vi "DancingLED.vi"() -> ()   [LabVIEW 2020]
uses:
  DancingLEDEnum.ctl
  bcbb1c2d-c491-4427-a344-9a07431e1d3e.vi
  939999a5-51db-4c4a-bf67-1753f00f95a7.vi
  fbb08f2d-998a-4061-bdb6-f44989c1556d.vi
  5b1967e0-138d-40db-84bc-8d854150fb75.vi
  e170c4a2-dbbe-475a-b394-96526eb2ee03.vi
  <vilib>/ErrorRing/Error Ring.xnode
panel:
  out "5":bool[](array[boolean])
  out "4":bool[](array[boolean])
  out "3":bool[](array[boolean])
  out "2":bool[](array[boolean])
  out "1":bool[](array[boolean])
  in  "Switch":bool
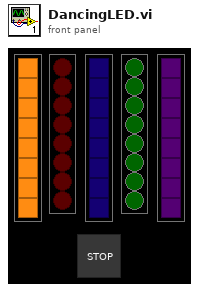
[diagram p1: front panel]
types:
  T1 = typedef "DancingLEDEnum.ctl" = enum16{"IDLE", "CONTROL", "UIInit", "DataUpdate", "UPDATE", "EXIT"}
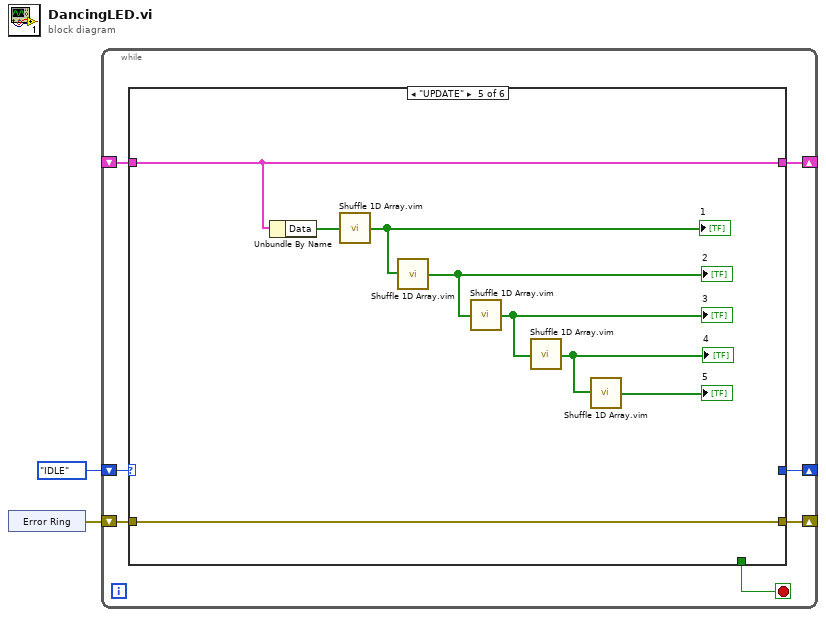
[diagram p0: block diagram]
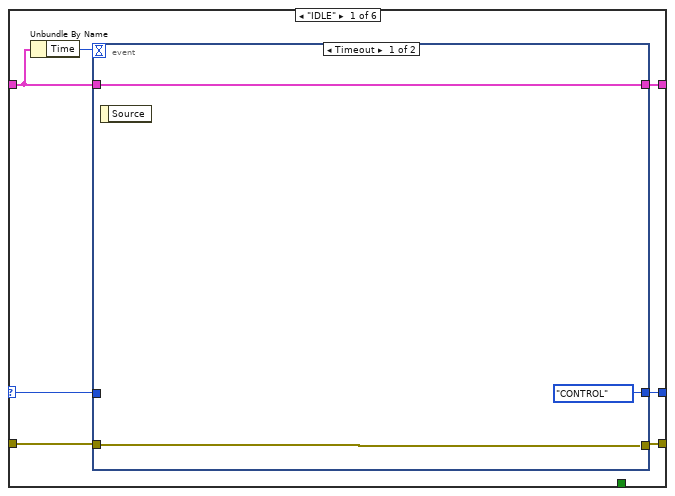
[diagram p2: hidden frame]
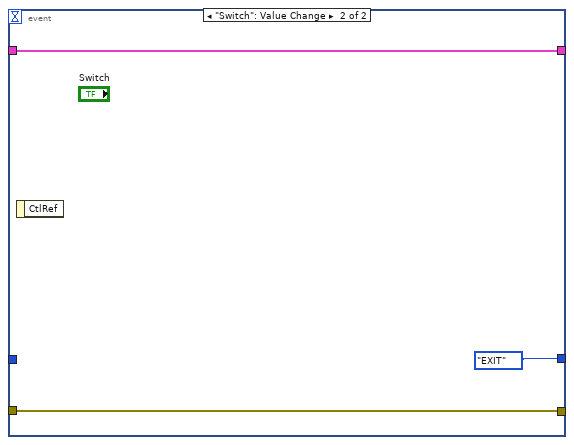
[diagram p3: hidden frame]
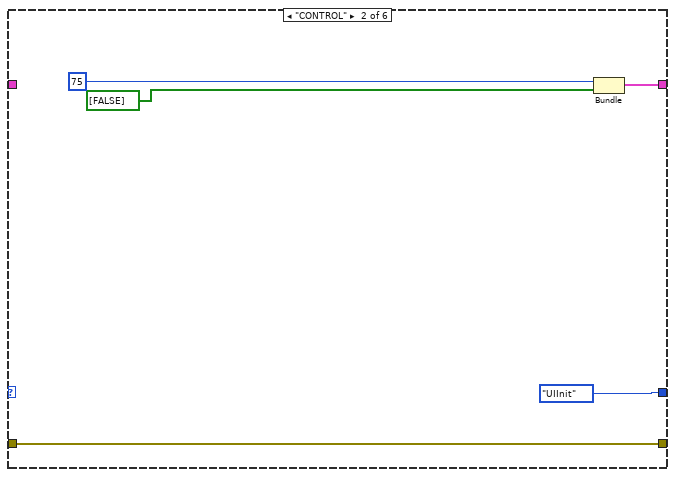
[diagram p4: hidden frame]
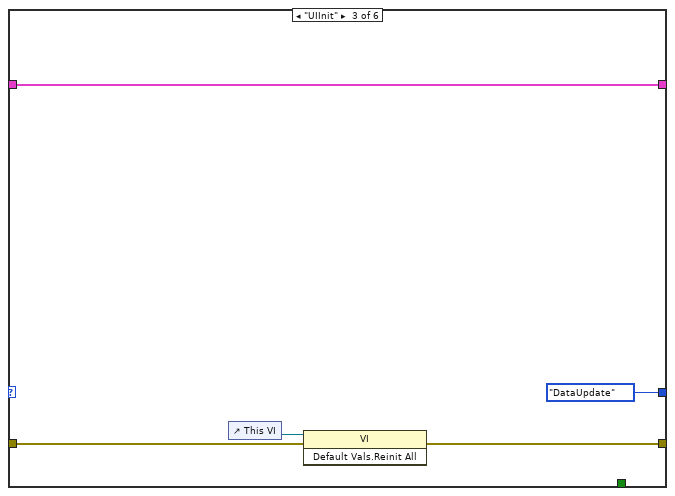
[diagram p5: hidden frame]
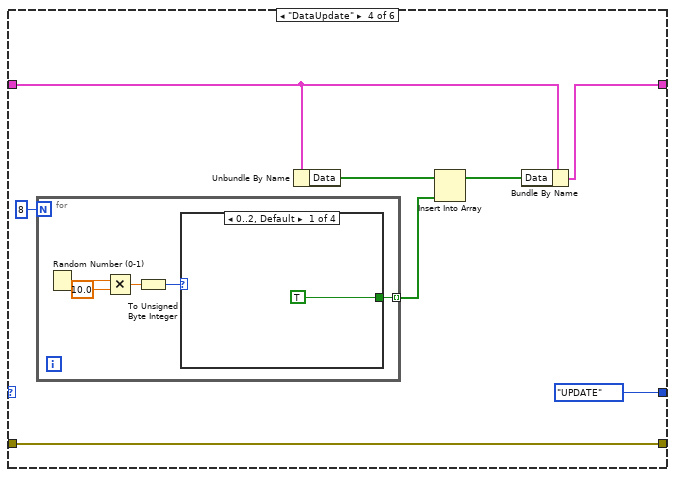
[diagram p6: hidden frame]
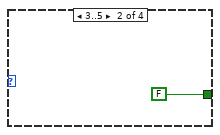
[diagram p7: hidden frame]
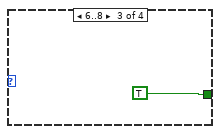
[diagram p8: hidden frame]
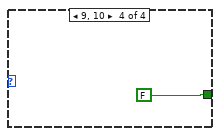
[diagram p9: hidden frame]
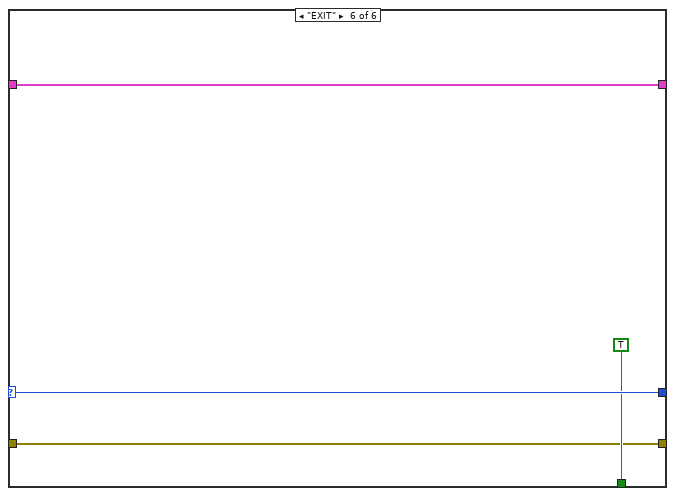
[diagram p10: hidden frame]
diagram:
  n1 = xnode "Error Ring"() -> ("error out"=w1:errorcluster)
  n2 = while {
    shift-right: [w5] -> _
    shift-left: _ -> [w6]
    shift-right: [w8] -> _
    shift-left: DancingLEDEnum."IDLE" -> [w9]
    shift-right: [w3] -> _
    shift-left: w1 -> [w4]
    stop <- w7 stop-if-true
    n3 = case shown="\"UPDATE\"" w9 {
      selector: w9 -> [w16 _ _ _ _ w61]
      tunnel: [w15 DancingLEDEnum."UIInit" DancingLEDEnum."DataUpdate" DancingLEDEnum."UPDATE" _ w61] -> w8
      tunnel: [_ _ _ _ _ TRUE] -> w7
      tunnel: w6 -> [w11 _ w32 w36 w52 w59]
      tunnel: [w14 w25 w32 w39 w52 w59] -> w5
      tunnel: w4 -> [w13 w27 w30 w40 w57 w58]
      tunnel: [w12 w27 w29 w40 w57 w58] -> w3
      frame "IDLE" {
        n4 = Unbundle By Name(w11) -> ("Time"=w10:i32)
        n5 = event shown="[0] Timeout" {
          selector: _ -> [_ _]
          dyn-events: _ -> [_ _]
          timeout: w10 -> [_ _]
          tunnel: w16 -> [_ _]
          tunnel: [DancingLEDEnum."CONTROL" DancingLEDEnum."EXIT"] -> w15
          tunnel: w11 -> [w19 w21]
          tunnel: [w19 w21] -> w14
          tunnel: w13 -> [w17 w20]
          tunnel: [w17 w20] -> w12
          event Timeout {
            n6 = event-data() -> ()  [unwired: 1 in, 1 out]
          }
          event "Switch": Value Change {
            n7 = event-data() -> ()  [unwired: 1 in, 1 out]
          }
        }
      }
      frame "CONTROL" {
        n8 = Bundle("Time"=75, "Data"=bool[] [FALSE]) -> (w25:cluster{"Time":i32, "Data":bool[]})  [unwired: 1 in]
      }
      frame "UIInit" {
        n9 = control-ref of="This VI"() -> (w31:refnum<vi>)
        n10 = invoke class="VI" method="Default Vals.Reinit All"(reference=w31, error in=w30) -> (error out=w29:errorcluster)  [unwired: 1 in, 2 out]
      }
      frame "DataUpdate" {
        n11 = for {
          N: 8 -> [_]
          tunnel: [w41] -> w34 mode=indexing
          n12 = Random Number (0-1)() -> (number: 0 to 1=w44:dbl)
          n13 = Multiply(x=w44, y=10.0) -> (x*y=w42:dbl)
          n14 = To Unsigned Byte Integer(number=w42) -> (unsigned 8bit integer=w45:u8)
          n15 = case shown="0..2, Default" w45 {
            tunnel: [TRUE FALSE TRUE FALSE] -> w41
            frame 0..2, Default {
            }
            frame 3..5 {
            }
            frame 6..8 {
            }
            frame 9, 10 {
            }
          }
        }
        n16 = Unbundle By Name(w36) -> ("Data"=w35:bool[])
        n17 = Insert Into Array(array=w35, new element=w34) -> (w33:bool[])  [unwired: 1 in]
        n18 = Bundle By Name(cluster=w36, "Data"=w33) -> (w39:cluster{"Time":i32, "Data":bool[]})
      }
      frame "UPDATE" {
        n19 = Unbundle By Name(w52) -> ("Data"=w50:bool[])
        n20 = call "Shuffle 1D Array.vim"("array"=w50) -> ("shuffled array"=w51:bool[])  [unwired: 4 in]
        "1" <- w51
        n21 = call "Shuffle 1D Array.vim"("array"=w51) -> ("shuffled array"=w56:bool[])  [unwired: 4 in]
        "2" <- w56
        n22 = call "Shuffle 1D Array.vim"("array"=w56) -> ("shuffled array"=w55:bool[])  [unwired: 4 in]
        "3" <- w55
        n23 = call "Shuffle 1D Array.vim"("array"=w55) -> ("shuffled array"=w54:bool[])  [unwired: 4 in]
        "4" <- w54
        n24 = call "Shuffle 1D Array.vim"("array"=w54) -> ("shuffled array"=→"5":bool[])  [unwired: 4 in]
      }
      frame "EXIT" {
      }
    }
  }
